vi "FloaterCalc.vi"(0 "Log":bool, 1 "medians":i32=-1, 2 "left rank":i32=2, 3 "ROI Box":u16[](array[numeric]), 5 "Scan Info":T1 {"delay" format="%.2f"; "pivot distance" format="%.2f"; "sector scan angle" format="%.2f"}, 6 "new path in":path, 9 "Raw Data In":dbl[][](array[numeric])) -> (15 "Masked Data":dbl[][](graph), 19 "RMS noise x6":dbl format="%#.2g")   [LabVIEW 2022 SP3]
uses:
  <vilib>/Analysis/5stat.llb/RMS (DBL).vi
  <vilib>/Utility/file.llb/Write Delimited Spreadsheet (string).vi
  <vilib>/Analysis/NI_AALBase.lvlib
  <vilib>/Analysis/NI_AALPro.lvlib
panel:
  out "Sector":dbl[][](graph)
  out "Raw Mean filter Data Out":dbl[][](graph)
  out "mean above thresh":dbl
  out "pix above thresh":i32
  out "Dynamic Range":dbl
  out "Raw Data Out":dbl[][](graph)
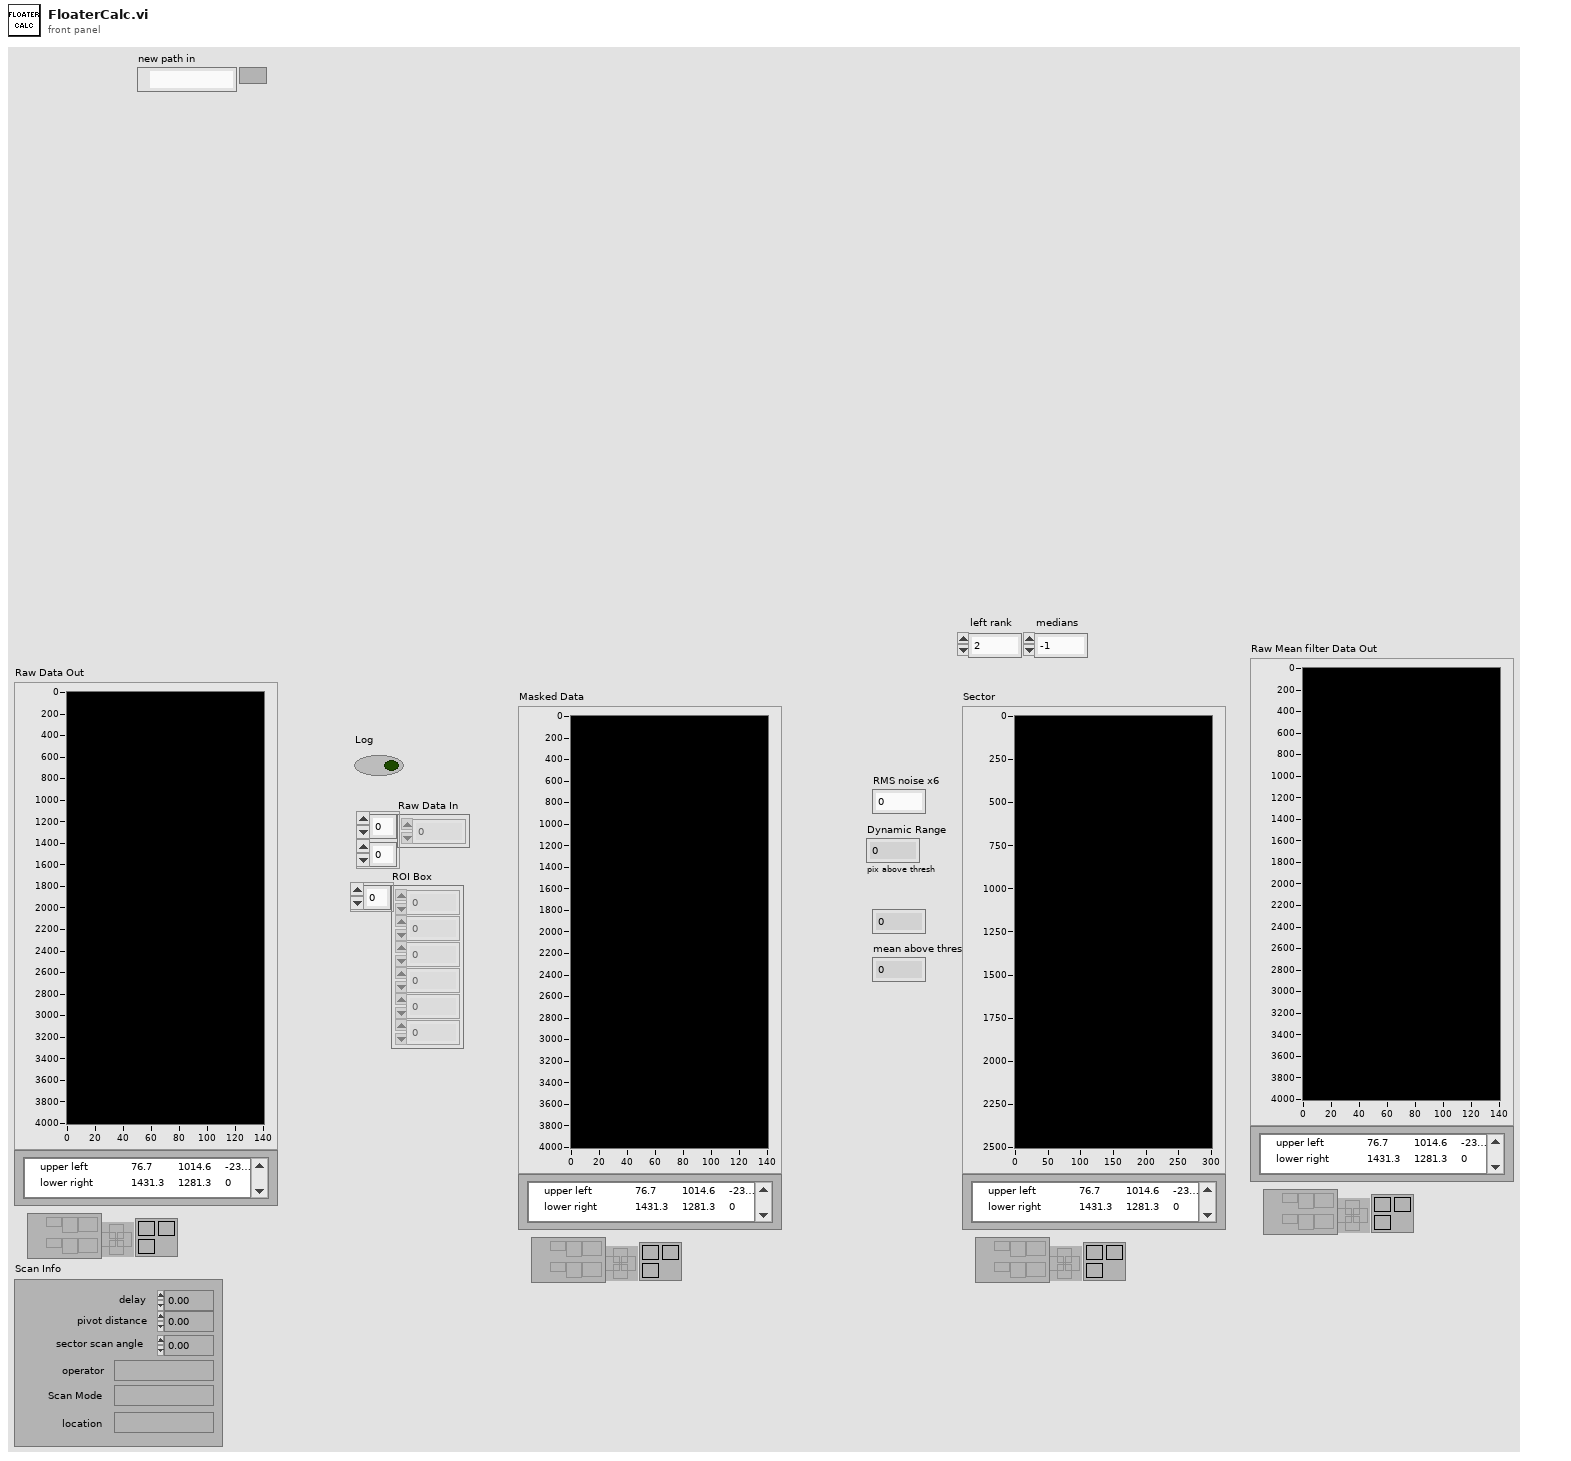
[diagram p1: front panel]
types:
  T1 = cluster{"delay":sgl, "pivot distance":sgl, "sector scan angle":sgl, "operator":string, "Scan Mode":string, "location":string}
  T2 = cluster{"ROI Box[0]":u16, "ROI Box[1]":u16, "ROI Box[2]":u16, "ROI Box[3]":u16}
  T3 = typedef "imagedata.ctl" = cluster{"image type":i32, "image depth":i32, "image":u8[], "mask":u8[], "colors":u32[], "Rectangle":cluster{"left":i16, "top":i16, "right":i16, "bottom":i16}}
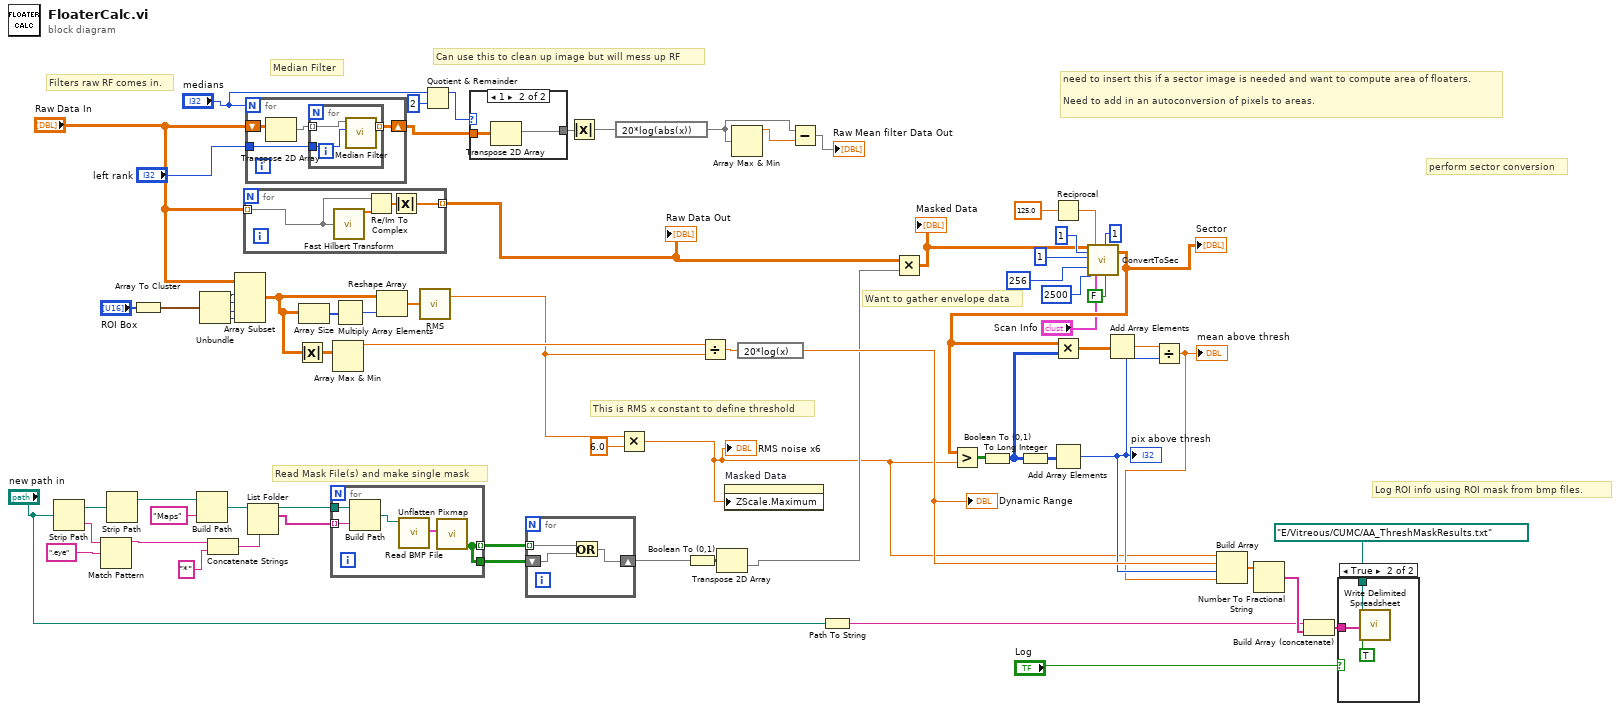
[diagram p0: block diagram]
diagram:
  # "Filters raw RF comes in."
  # "Want to gather envelope data"
  # "Can use this to clean up image but will mess up RF"
  # "Log ROI info using ROI mask from bmp files."
  # "need to insert this if a sector image is needed and want to compute area of floaters.\n\nNeed to add in an autoconversion of pixels to areas."
  # "perform sector conversion"
  # "This is RMS x constant to define threshold"
  # "Read Mask File(s) and make single mask"
  # "Median Filter"
  n1 = Strip Path(path="new path in") -> (stripped path=w63:path, name=w60:string)
  n2 = Match Pattern(string=w60, regular expression=".eye") -> (before substring=w62:string)  [unwired: 1 in, 3 out]
  n3 = Strip Path(path=w63) -> (stripped path=w64:path)  [unwired: 1 out]
  n4 = Array To Cluster(array="ROI Box") -> (cluster=w34:T2)
  n5 = Build Path(base path=w64, name or relative path="Maps") -> (appended path=w57:path)
  n6 = Unbundle(w34) -> ("ROI Box[0]"=w33:u16, "ROI Box[1]"=w32:u16, "ROI Box[2]"=w31:u16, "ROI Box[3]"=w30:u16)
  n7 = Concatenate Strings(w62, "*" ("pattern")) -> (w59:string)
  n8 = Array Subset(array="Raw Data In", index (row)=w33, length (row)=w32, index (col)=w31, length (col)=w30) -> (w19:dbl[][])
  n9 = for {
    tunnel: "Raw Data In" -> [w72] mode=indexing
    tunnel: [w71] -> w24 mode=indexing
    n10 = call <vilib>:"Fast Hilbert Transform.vi"("X"=w72) -> ("Hilbert{X}"=w73:dbl[])  [unwired: 1 out]
    n11 = Re/Im To Complex(1:w73, 2:w72) -> (0:w74:cdb[])
    n12 = Absolute Value(x=w74) -> (abs(x)=w71:dbl[])
  }
  "Raw Data Out" <- w24
  n13 = for {
    N: "medians" -> [_]
    shift-right: [w78] -> w54
    shift-left: "Raw Data In" -> [w77]
    tunnel: "left rank" -> [w76]
    n14 = Transpose 2D Array(2D array=w77) -> (transposed array=w75:dbl[][])
    n15 = for {
      tunnel: [w81] -> w78 mode=indexing
      tunnel: w76 -> [w80]
      tunnel: w75 -> [w79] mode=indexing
      n16 = call <vilib>:"Median Filter.vi"("left rank"=w80, "X"=w79) -> ("Filtered X"=w81:dbl[])  [unwired: 8 in, 1 out]
    }
  }
  n17 = List Folder(path=w57, pattern=w59) -> (path out=w65:path, filenames=w66:string[])  [unwired: 2 in, 2 out]
  n18 = Absolute Value(x=w19) -> (abs(x)=w20:dbl[][])
  n19 = Array Size(array=w19) -> (size(s)=w29:i32[])
  n20 = for {
    tunnel: w65 -> [w85]
    tunnel: w66 -> [w84] mode=indexing
    tunnel: [w82] -> w67 mode=indexing
    tunnel: [w82] -> w68
    n21 = Build Path(base path=w85, name or relative path=w84) -> (appended path=w83:path)
    n22 = call <vilib>:"Read BMP File.vi"("path to BMP file"=w83) -> ("image data"=w86:T3)  [unwired: 8 in, 2 out]
    n23 = call <vilib>:"Unflatten Pixmap.vi"("image data"=w86) -> ("1-bit pixmap"=w82:bool[][])  [unwired: 4 in, 6 out]
  }
  n24 = Array Max & Min(array=w20) -> (max value=w18:dbl)  [unwired: 3 out]
  n25 = Multiply Array Elements(1:w29) -> (0:w27:i32)
  n26 = Reshape Array(w19, w27) -> (w28:dbl[])
  n27 = call-poly <vilib>:"RMS.vi"("X"=w28) -> ("rms value"=w1:dbl)  [unwired: 1 out]
  n28 = Quotient & Remainder(x="medians", y=2) -> (x-y*floor(x/y)=w55:i32)  [unwired: 1 out]
  n29 = case shown="1" w55 {
    tunnel: w54 -> [w87 w89]
    tunnel: [w87 w88] -> w70
    frame 0, Default {
    }
    frame 1 {
      n30 = Transpose 2D Array(2D array=w89) -> (transposed array=w88:dbl[][])
    }
  }
  n31 = for {
    tunnel: w67 -> [w92] mode=indexing
    shift-right: [w91] -> w69
    shift-left: w68 -> [w90]
    n32 = Or(x=w92, y=w90) -> (x .or. y?=w91:bool[][])
  }
  n33 = Absolute Value(x=w70) -> (abs(x)=w15:dbl[][])
  n34 = expression code="20*log(abs(x))"(w15) -> (w14:dbl[][])
  n35 = Multiply(x=w1, y=6.0) -> (x*y=w22:dbl)
  "RMS noise x6" <- w22
  n36 = Boolean To (0,1)(Boolean=w69) -> (0, 1=w26:i16[][])
  n37 = Divide(x=w18, y=w1) -> (x/y=w47:dbl)
  n38 = Transpose 2D Array(2D array=w26) -> (transposed array=w23:i16[][])
  n39 = property on="Masked Data" class="IntGraph (strict)"("ZScale.Maximum"=w22) -> ()  [unwired: 2 in, 2 out]
  n40 = Array Max & Min(array=w14) -> (max value=w17:dbl)  [unwired: 3 out]
  n41 = expression code="20*log(x)"(w47) -> (w46:dbl)
  "Dynamic Range" <- w46
  n42 = Subtract(x=w14, y=w17) -> (x-y=→"Raw Mean filter Data Out":dbl[][])
  n43 = Path To String(path="new path in") -> (string=w41:string)
  n44 = Multiply(x=w24, y=w23) -> (x*y=w4:dbl[][])
  "Masked Data" <- w4
  n45 = Reciprocal(x=125.0) -> (1/x=w13:dbl)
  n46 = call "ConvertToSec.vi"("raw image data in"=w4, "reduce pts by factor of"=1 ("Reduce x data factor"), "Add Lines"=u16 1, "pixels in x"=i16 256 ("Pixels in x"), "pixels in y"=i16 2500 ("Pixels in y"), "Time between rf pts\nmicros"=w13, "Scan Info"="Scan Info", "Smooth factor"=1, "use min z value?"=FALSE) -> ("raw sector out"=w3:dbl[][])  [unwired: 3 in, 7 out]
  "Sector" <- w3
  n47 = Greater?(x=w3, y=w22) -> (0:w50:bool[][])
  n48 = Boolean To (0,1)(Boolean=w50) -> (0, 1=w39:i16[][])
  n49 = To Long Integer(number=w39) -> (32bit integer=w49:i32[][])
  n50 = Multiply(x=w3, y=w39) -> (x*y=w7:dbl[][])
  n51 = Add Array Elements(numeric array=w49) -> (sum=w37:i32)
  "pix above thresh" <- w37
  n52 = Add Array Elements(numeric array=w7) -> (sum=w38:dbl)
  n53 = Divide(x=w38, y=w37) -> (x/y=w36:dbl)
  "mean above thresh" <- w36
  n54 = Build Array(w22, w46, w37, w36) -> (w45:dbl[])
  n55 = Number To Fractional String(number=w45) -> (F-format string=w42:string[])  [unwired: 3 in]
  n56 = Build Array (concatenate)(w41, w42) -> (w44:string[])
  n57 = case shown="True" "Log" {
    tunnel: w44 -> [_ w95]
    tunnel: path "E:/Vitreous/CUMC/AA_ThreshMaskResults.txt" ("file path (dialog if empty)") -> [_ w94]
    frame False {
    }
    frame True {
      n58 = call-poly <vilib>:"Write Delimited Spreadsheet.vi"("file path (dialog if empty)"=w94, "1D data"=w95, "append to file? (new file:F)"=TRUE ("append to file? (F)")) -> ()  [unwired: 11 in, 2 out]
    }
  }
